vi "I2C Host Test.vi"() -> ()   [LabVIEW 2012]
uses:
  <vilib>/Platform/TimedLoop/XDataNode/timing_clust.ctl
  <vilib>/Platform/TimedLoop/XDataNode/nitl_modes.ctl
  <vilib>/Platform/TimedLoop/XDataNode/wakeup.ctl
  <vilib>/FPGAPlugInAG/sbRIO-9636/niLvFpga_Open_sbRIO-9636.vi
  <vilib>/rvi/interface/common/dynamic/niFpgaDynamicAddResources.vi
  <vilib>/FPGAPlugInAG/Dynamic/niLvFpga_Close_Dynamic.vi
  <vilib>/platform/TimedLoop/XDataNode/XDataNode.xnode
  <vilib>/rvi/interface/nirviOpenFPGA/nirviOpenFPGA.xnode
  FPGA Bitfiles/NIARC_FPGATarget_FPGACompile_e4XhunWUay0.lvbitx
  <vilib>/rvi/interface/nirviCloseFPGA/nirviCloseFPGA.xnode
  <vilib>/Platform/TimedLoop/XDataNode/XDNodeRunTimeDep.lvlib
  <vilib>/IEDriver/SPIandI2C/Host/I2C/I2C Host.lvlib
panel:
  in  "Clock Rate":u32=1000
  in  "stop":bool
  in  "Address Type (7-bit)":enum16{"7-bit", "10-bit"}(ring)
  in  "FPGA Clock (40 MHz)":u32=40000000
  in  "Port Number":u8
  in  "Address":u16=25 format="%.0x"
  in  "Write Data":u8[](array[numeric])=[80] format="%.0x"
  in  "Timeout (10 s)":u8=10
  out "Read Data":u8[](array[numeric])
  out "32bit integer":i32
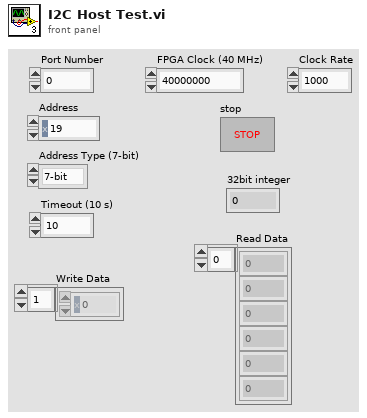
[diagram p1: front panel]
types:
  T1 = typedef "XDNodeRunTimeDep.lvlib/timing_clust.ctl" = cluster{"Expected End [f-1]":u64, "Actual End [f-1]":u64, "Finished Late? [f-1]":bool, "Expected End [i-1]":u64, "Actual End [i-1]":u64, "Finished Late? [i-1]":bool, "Expected Start [i]":u64, "Actual Start [i]":u64, "Expected Start [f]":u64, "Actual Start [f]":u64, "Source Name":string, "Structure Name":string, "Period":i64, "Deadline":i64, "Offset":i64, "Start":i64, "Priority":i32, "Timeout":i32, "Mode":T2, "Wakeup Reason":T3, "Error":errorcluster, "Source Type":string, "Secondary Source Type":string, "Global End Time":u64, "Global Start Time":u64, "Frame Duration":u64, "Iteration Duration":u64, "Assigned CPU":i32, "I/O Scan Engine Mode":u32}
  T2 = typedef "XDNodeRunTimeDep.lvlib/nitl_modes.ctl" = enum32{"No Change", "Process missed periods, maintain original phase", "Discard missed periods, maintain original phase", "Process missed periods, ignore original phase", "Discard missed periods, ignore original phase"}
  T3 = typedef "XDNodeRunTimeDep.lvlib/wakeup.ctl" = enum32{"Normal", "Aborted", "Asynchronous wakeup", "Timing source error", "Timed loop error", "Timeout"}
  T4 = cluster{"FPGA VI Reference":refnum<k20>, "Port Number":u8}
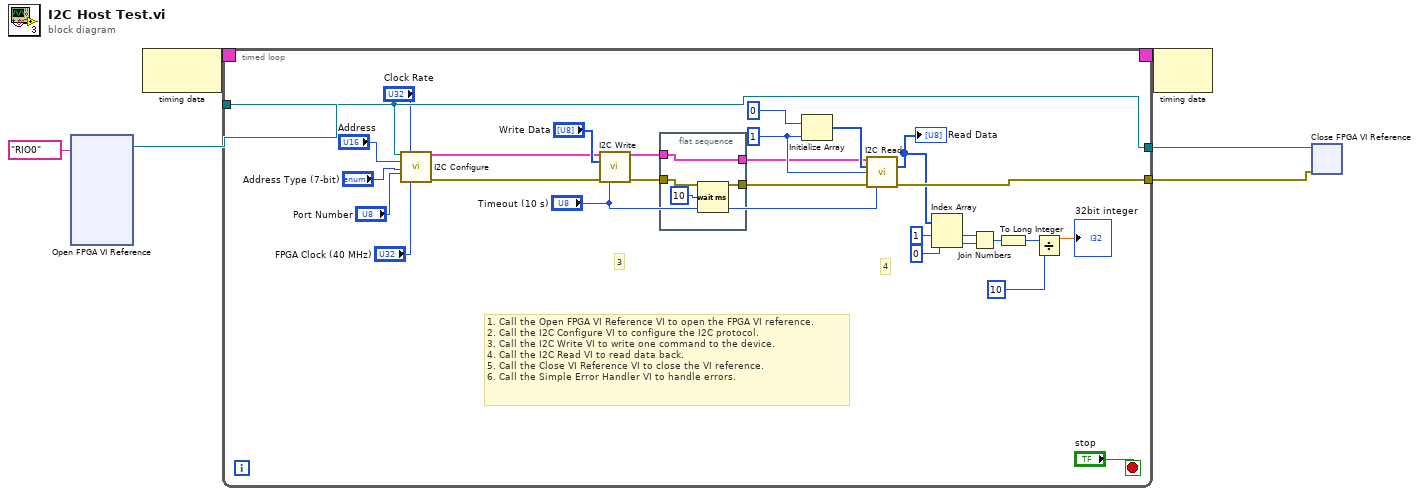
[diagram p0: block diagram]
diagram:
  n1 = xnode "Open FPGA VI Reference"("resource name"=tag "RIO0") -> ("FPGA VI Reference Out"=w2:refnum<k20>)  [unwired: 1 in, 1 out]
  n2 = node-c288() -> (w6:T1)  [unwired: 1 in]
  n3 = timed-loop {
    timing: w6 -> [_]
    timing-out: [_] -> w5
    tunnel: [w34] -> w4
    tunnel: w2 -> [w14]
    tunnel: [w14] -> w1
    stop <- "stop" stop-if-true
    w31 = u16 1 ("Number of Bytes to Read")
    # "1. Call the Open FPGA VI Reference VI to open the FPGA VI reference.\n2. Call the I2C Configure VI to configure the I2C protocol.\n3. Call the I2C Write VI to write one command to the device.\n4. Call the I2C Read VI to read data back.\n5. Call the Close VI Reference VI to close the VI reference.\n6. Call the Simple Error Handler VI to handle errors."
    # "4"
    # "3"
    n4 = call <vilib>:"I2C Configure.vi"("FPGA VI Reference"=w14, "Clock Rate"="Clock Rate", "Address"="Address", "Address Type (7-bit)"="Address Type (7-bit)", "Port Number"="Port Number", "FPGA Clock (40 MHz)"="FPGA Clock (40 MHz)") -> ("FPGA Information Out"=w13:T4, "error out"=w12:errorcluster)  [unwired: 8 in]
    n5 = call <vilib>:"I2C Write.vi"("FPGA Information In"=w13, "Data"="Write Data", "error in (no error)"=w12, "Timeout (10 s)"="Timeout (10 s)") -> ("FPGA Information Out"=w21:T4, "error out"=w20:errorcluster)  [unwired: 10 in]
    n6 = flat-sequence {
      tunnel: w21 -> [w37]
      tunnel: w20 -> [w36]
      tunnel: [w37] -> w19
      tunnel: [w36] -> w18
      frame #0 {
        n7 = Wait (ms)(milliseconds to wait=u32 10) -> ()  [unwired: 1 out]
      }
    }
    n8 = Initialize Array(u8 0, w31) -> (w29:u8[])
    n9 = call <vilib>:"I2C Read.vi"("FPGA Information In"=w19, "Input Array"=w29, "Number of Bytes to Read"=w31, "error in (no error)"=w18, "Timeout (10 s)"="Timeout (10 s)") -> ("Data"=w28:u8[], "error out"=w34:errorcluster)  [unwired: 8 in, 1 out]
    "Read Data" <- w28
    n10 = Index Array(array=w28, index #1=1 ("index"), index #2=0 ("index")) -> (element #1=w26:u8, element #2=w27:u8)
    n11 = Join Numbers(hi=w26, lo=w27) -> ((hi.lo)=w25:u16)
    n12 = To Long Integer(number=w25) -> (32bit integer=w22:i32)
    n13 = Divide(x=w22, y=10) -> (x/y=→"32bit integer":dbl)
  }
  n14 = node-c288(w5) -> ()  [unwired: 1 out]
  n15 = xnode "Close FPGA VI Reference"("FPGA VI Reference In"=w1, "error in"=w4) -> ()  [unwired: 1 out]
